vi "Find 007.vi"(8 "Error In":errorcluster, 11 "Player Names":string[](array[string])) -> (0 "Error Out":errorcluster, 3 "007 Data":T1)   [LabVIEW 2015]
uses:
  007 Data.ctl
panel:
  in  "007 Data 2":T1
  out "id Mandingo":dbl
  out "Found 007":bool
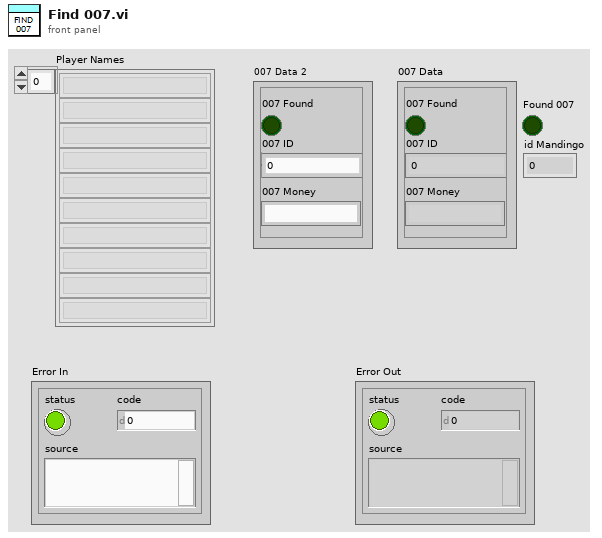
[diagram p1: front panel]
types:
  T1 = typedef "007 Data.ctl" = cluster{"007 ID":dbl, "007 Found":bool, "007 Money":string}
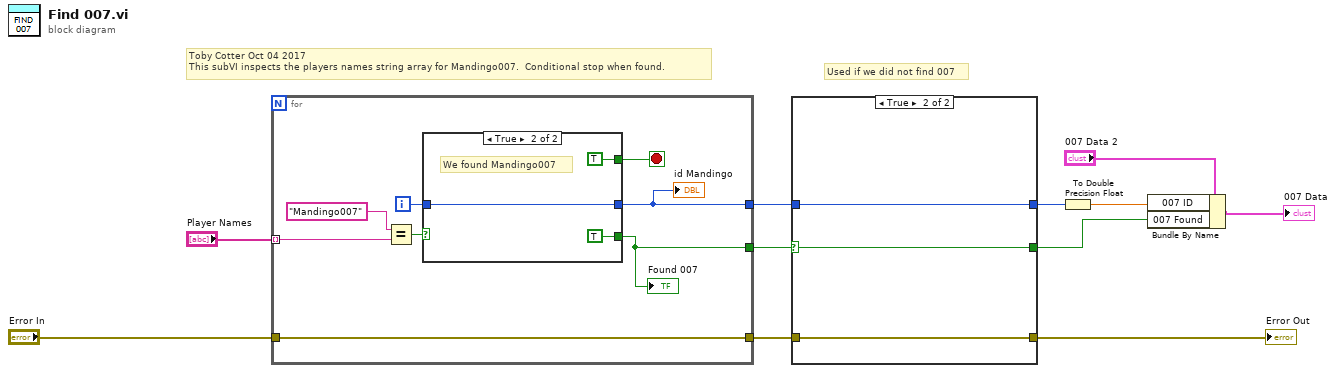
[diagram p0: block diagram]
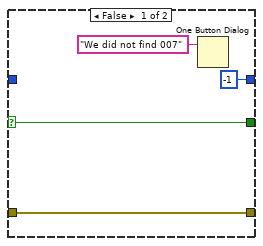
[diagram p2: hidden frame]
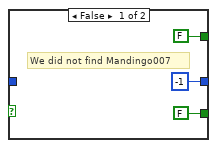
[diagram p3: hidden frame]
diagram:
  # "Used if we did not find 007"
  # "Toby Cotter Oct 04 2017\nThis subVI inspects the players names string array for Mandingo007.  Conditional stop when found."
  n1 = for {
    tunnel: "Player Names" -> [w19] mode=indexing
    tunnel: "Error In" -> [w14]
    tunnel: [w14] -> w9
    tunnel: [w13] -> w7
    tunnel: [w12] -> w6
    i -> [w16]
    stop <- w15 stop-if-true
    n2 = Equal?(x="Mandingo007", y=w19) -> (x = y?=w17:bool)
    n3 = case shown="True" w17 {
      tunnel: [FALSE ("Found Mandingo") TRUE ("Found Mandingo")] -> w13
      tunnel: w16 -> [_ w23]
      tunnel: [-1 w23] -> w12
      tunnel: [FALSE ("Found Mandingo") TRUE ("Found Mandingo")] -> w15
      frame False {
        # "We did not find Mandingo007"
      }
      frame True {
        # "We found Mandingo007"
      }
    }
    "Found 007" <- w13
    "id Mandingo" <- w12
  }
  n4 = case shown="True" w7 {
    selector: w7 -> [w27 w30]
    tunnel: [w29 w32] -> w8
    tunnel: w9 -> [w29 w32]
    tunnel: [w27 w30] -> w2
    tunnel: w6 -> [_ w31]
    tunnel: [-1 w31] -> w3
    frame False {
      n5 = One Button Dialog(message="We did not find 007") -> ()  [unwired: 1 in, 1 out]
    }
    frame True {
    }
  }
  "Error Out" <- w8
  n6 = To Double Precision Float(number=w3) -> (double precision float=w4:dbl)
  n7 = Bundle By Name(cluster="007 Data 2", "007 ID"=w4, "007 Found"=w2) -> (→"007 Data":T1)
